vi "Problem 8 - Largest product in a series.vi"() -> (3 "Answer":dbl format="%#.1f")   [LabVIEW 2021, in "Project Euler.lvlib"]
uses:
  Project Euler.lvlib
panel:
  out "no. of groups of adjacent digits":i32
  in  "no. of adjacent digits":i32=13
  out "input string length":i32
  in  "1000-digit number":string="7316717653133062491922511967442657474235534919493496983520312774506326239578318016984801869478851843858615607891129494954595017379583319528532088055111254069874715852386305071569329096329522744304355766896648950445244523161731856403098711121722383113622298934233803081353362766142828064444866452387493035890729629049156044077239071381051585930796086670172427121883998797908792274921901699720888093776657273330010533678812202354218097512545405947522435258490771167055601360483958644670632441572215539753697817977846174064955149290862569321978468622482839722413756570560574902614079729686524145351004748216637048440319989000889524345065854122758866688116427171479924442928230863465674813919123162824586178664583591245665294765456828489128831426076900422421902267105562632111110937054421750694165896040807198403850962455444362981230987879927244284909188845801561660979191338754992005240636899125607176060588611646710940507754100225698315520005593572972571636269561882670428252483600823257530420752963450"
  # "Development\nControls or indicators that are useful for development or testing, but which are not outputs of the VI."
  # "Input\nInputs to the VI"
  # "Output\nOutputs of the VI"
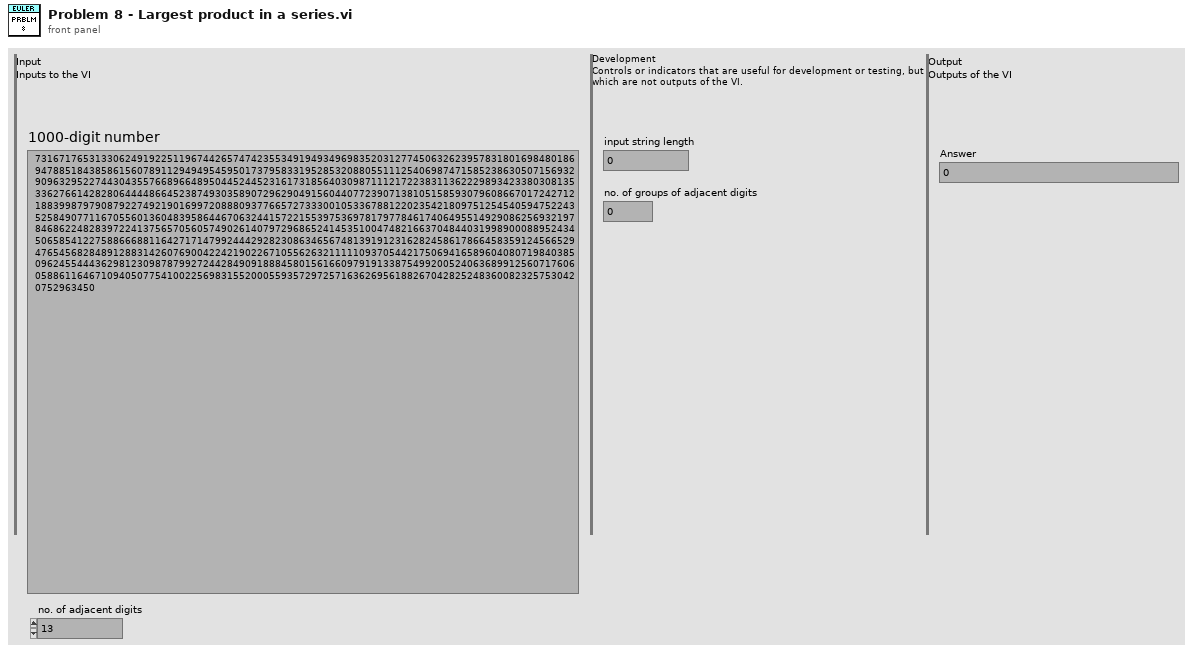
[diagram p1: front panel]
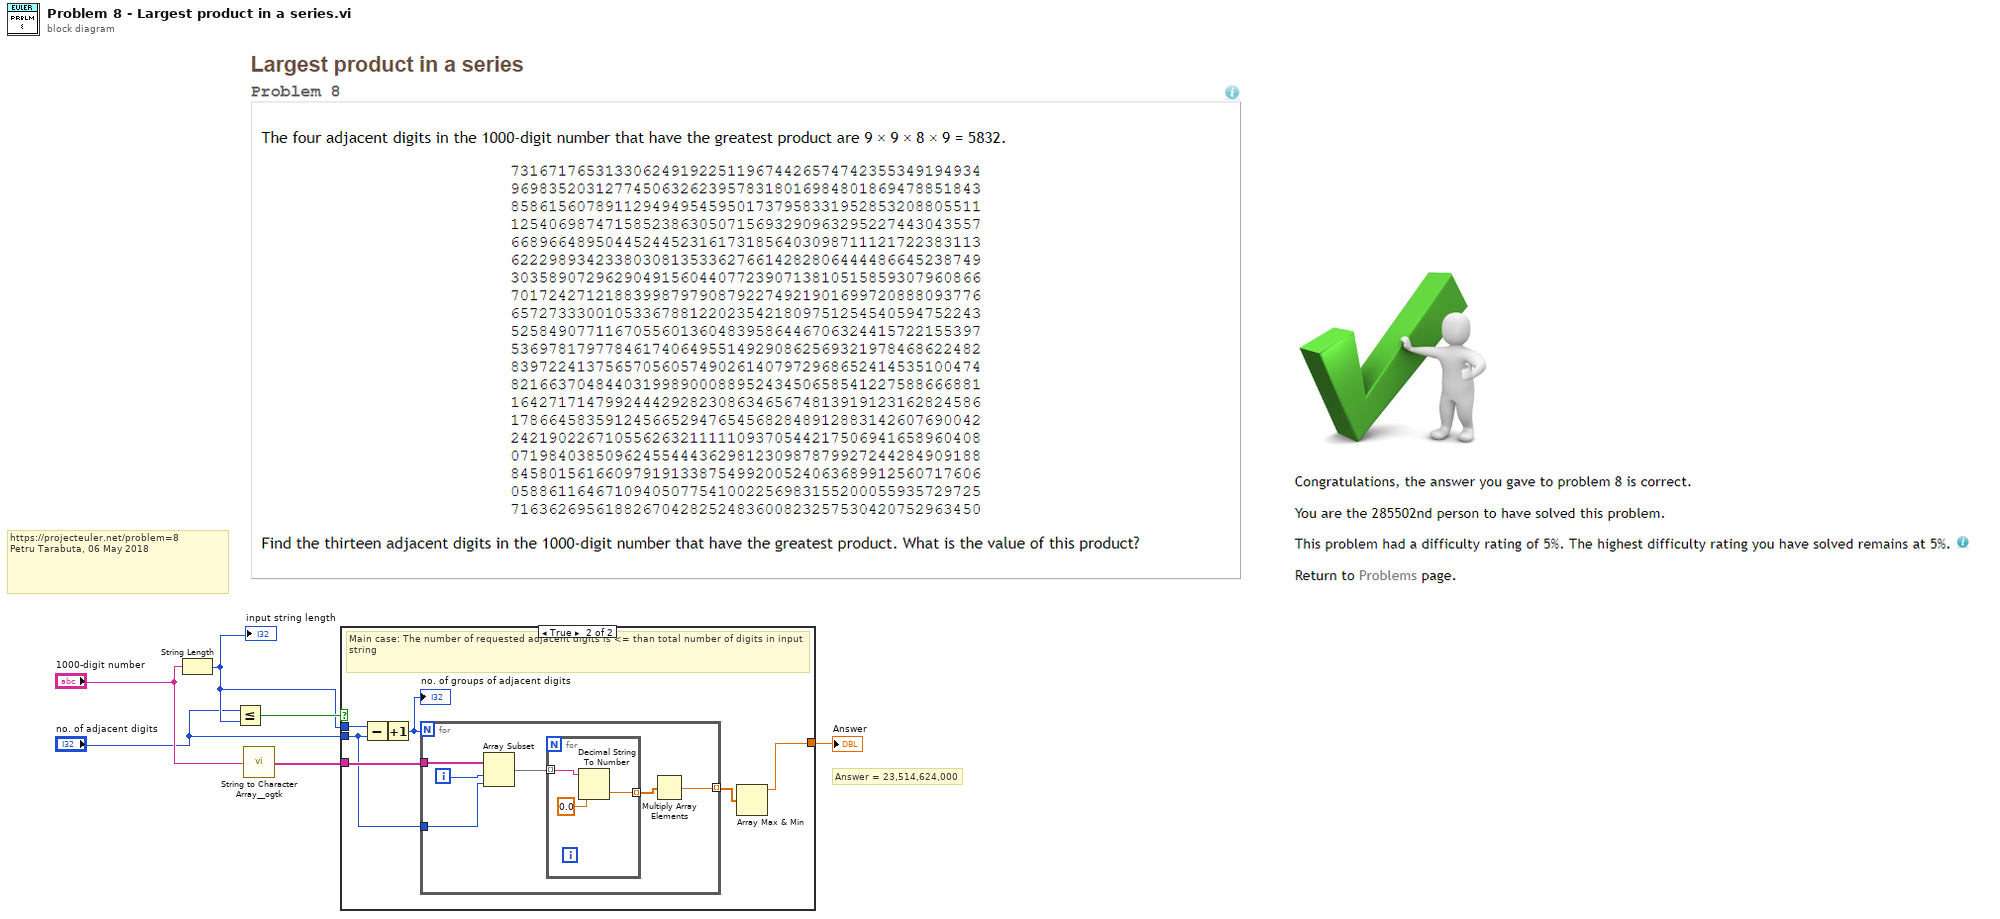
[diagram p0: block diagram]
diagram:
  # "Answer = 23,514,624,000"
  # "https://projecteuler.net/problem=8\nPetru Tarabuta, 06 May 2018"
  n1 = String Length(string="1000-digit number") -> (length=w3:i32)
  "input string length" <- w3
  n2 = Less Or Equal?(x="no. of adjacent digits", y=w3) -> (x <= y?=w6:bool)
  n3 = call <userlib>:"String to Character Array__ogtk.vi"("Input String"="1000-digit number") -> ("Character Array"=w1:string[])
  n4 = case shown="True" w6 {
    tunnel: [_ w8] -> w5
    tunnel: w1 -> [_ w11]
    tunnel: w3 -> [_ w13]
    tunnel: "no. of adjacent digits" -> [_ w10]
    frame False {
      # "Corner case"
    }
    frame True {
      # "Main case: The number of requested adjacent digits is <= than total number of digits in input string"
      n5 = Subtract(x=w13, y=w10) -> (x-y=w12:i32)
      n6 = Increment(x=w12) -> (x+1=w7:i32)
      "no. of groups of adjacent digits" <- w7
      n7 = for {
        N: w7 -> [_]
        tunnel: w11 -> [w19]
        tunnel: w10 -> [w17]
        tunnel: [w14] -> w9 mode=indexing
        i -> [w18]
        n8 = Array Subset(array=w19, index=w18, length=w17) -> (w16:string[])
        n9 = for {
          tunnel: w16 -> [w22] mode=indexing
          tunnel: [w21] -> w15 mode=indexing
          n10 = Decimal String To Number(string=w22, default (0L)=0.0) -> (number=w21:dbl)  [unwired: 1 in, 1 out]
        }
        n11 = Multiply Array Elements(1:w15) -> (0:w14:dbl)
      }
      n12 = Array Max & Min(array=w9) -> (max value=w8:dbl)  [unwired: 3 out]
    }
  }
  "Answer" <- w5
